vi "track_event.read.vi"(8 "error in":errorcluster, 11 "Track Chunk Core":u8[](array[numeric])) -> (0 "error out":errorcluster, 2 "file events":refnum<class "midi-file-event.lvclass">[](array[class]), 3 "Track Chunk Core Out":u8[](array[numeric]))   [LabVIEW 2020, in "midi-file.lvclass"]
uses:
  midi-file.lvclass
  midi-file-event/midi-file-event.lvclass
  MIDI Meta Events.ctl
  midi-file-event.meta/midi-file-event.meta.lvclass
  C:/code/LabVIEW-MIDI/lv-src/midi-file-event/midi-file-event.lvclass
  midi-file-event.meta/midi-file-event.meta.lvclass/midi-file-event.meta.ctl
  MIDI Messages.ctl
  midi-file-event.midi/midi-file-event.midi.lvclass
  midi-file-event.midi/midi-file-event.midi.lvclass/midi-file-event.midi.ctl
  midi-file-event/midi-file-event.lvclass/midi-file-event.ctl
  midi-file-event.meta/status.set.vi
  midi-file-event.meta/numeric_data.set.vi
  midi-file-event.meta/string_data.set.vi
  midi-file-event.midi/MIDI Messages.set.vi
  midi-file-event.midi/Data1.set.vi
  midi-file-event.midi/Data2.set.vi
  midi-file-event/Delta Tiime.set.vi
  midi-file-event/uid.set.vi
  midi-file.lvclass/midi-file.ctl
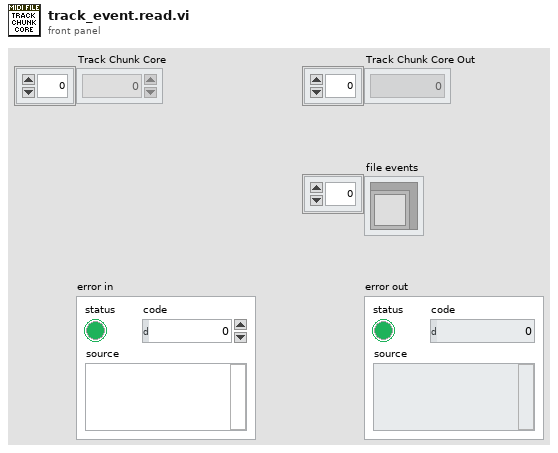
[diagram p1: front panel]
types:
  T1 = typedef "midi-file.lvclass/MIDI Meta Events.ctl" = enum8{"0(0x00)_SequenceNumber", "1(0x01)_TextEvent", "2(0x02)_CopyrightNotice", "3(0x03)_TrackOrSequenceName", "4(0x04)_InstrumentName", "5(0x05)_LyricText", "6(0x06)_MarkerText", "7(0x07)_CuePoint", "8(0x08)_UnassignedMetaEvent", "9(0x09)_UnassignedMetaEvent", "10(0x0A)_UnassignedMetaEvent", "11(0x0B)_UnassignedMetaEvent", "12(0x0C)_UnassignedMetaEvent", "13(0x0D)_UnassignedMetaEvent", "14(0x0E)_UnassignedMetaEvent", "15(0x0F)_UnassignedMetaEvent", "16(0x10)_UnassignedMetaEvent", "17(0x11)_UnassignedMetaEvent", "18(0x12)_UnassignedMetaEvent", "19(0x13)_UnassignedMetaEvent", "20(0x14)_UnassignedMetaEvent", "21(0x15)_UnassignedMetaEvent", "22(0x16)_UnassignedMetaEvent", "23(0x17)_UnassignedMetaEvent", "24(0x18)_UnassignedMetaEvent", "25(0x19)_UnassignedMetaEvent", "26(0x1A)_UnassignedMetaEvent", "27(0x1B)_UnassignedMetaEvent", "28(0x1C)_UnassignedMetaEvent", "29(0x1D)_UnassignedMetaEvent", "30(0x1E)_UnassignedMetaEvent", "31(0x1F)_UnassignedMetaEvent", "32(0x20)_MidiChannelPrefix", "33(0x21)_UnassignedMetaEvent", "34(0x22)_UnassignedMetaEvent", "35(0x23)_UnassignedMetaEvent", "36(0x24)_UnassignedMetaEvent", "37(0x25)_UnassignedMetaEvent", "38(0x26)_UnassignedMetaEvent", "39(0x27)_UnassignedMetaEvent", "40(0x28)_UnassignedMetaEvent", "41(0x29)_UnassignedMetaEvent", "42(0x2A)_UnassignedMetaEvent", "43(0x2B)_UnassignedMetaEvent", "44(0x2C)_UnassignedMetaEvent", "45(0x2D)_UnassignedMetaEvent", "46(0x2E)_UnassignedMetaEvent", "47(0x2F)_EndOfTrack", "48(0x30)_UnassignedMetaEvent", "49(0x31)_UnassignedMetaEvent", "50(0x32)_UnassignedMetaEvent", "51(0x33)_UnassignedMetaEvent", "52(0x34)_UnassignedMetaEvent", "53(0x35)_UnassignedMetaEvent", "54(0x36)_UnassignedMetaEvent", "55(0x37)_UnassignedMetaEvent", "56(0x38)_UnassignedMetaEvent", "57(0x39)_UnassignedMetaEvent", "58(0x3A)_UnassignedMetaEvent", "59(0x3B)_UnassignedMetaEvent", "60(0x3C)_UnassignedMetaEvent", "61(0x3D)_UnassignedMetaEvent", "62(0x3E)_UnassignedMetaEvent", "63(0x3F)_UnassignedMetaEvent", "64(0x40)_UnassignedMetaEvent", "65(0x41)_UnassignedMetaEvent", "66(0x42)_UnassignedMetaEvent", "67(0x43)_UnassignedMetaEvent", "68(0x44)_UnassignedMetaEvent", "69(0x45)_UnassignedMetaEvent", "70(0x46)_UnassignedMetaEvent", "71(0x47)_UnassignedMetaEvent", "72(0x48)_UnassignedMetaEvent", "73(0x49)_UnassignedMetaEvent", "74(0x4A)_UnassignedMetaEvent", "75(0x4B)_UnassignedMetaEvent", "76(0x4C)_UnassignedMetaEvent", "77(0x4D)_UnassignedMetaEvent", "78(0x4E)_UnassignedMetaEvent", "79(0x4F)_UnassignedMetaEvent", "80(0x50)_UnassignedMetaEvent", "81(0x51)_TempoSetting", "82(0x52)_UnassignedMetaEvent", "83(0x53)_UnassignedMetaEvent", "84(0x54)_SMPTEOffset", "85(0x55)_UnassignedMetaEvent", "86(0x56)_UnassignedMetaEvent", "87(0x57)_UnassignedMetaEvent", "88(0x58)_TimeSignature", "89(0x59)_KeySignature", "90(0x5A)_UnassignedMetaEvent", "91(0x5B)_UnassignedMetaEvent", "92(0x5C)_UnassignedMetaEvent", "93(0x5D)_UnassignedMetaEvent", "94(0x5E)_UnassignedMetaEvent", "95(0x5F)_UnassignedMetaEvent", "96(0x60)_UnassignedMetaEvent", "97(0x61)_UnassignedMetaEvent", "98(0x62)_UnassignedMetaEvent", "99(0x63)_UnassignedMetaEvent", "100(0x64)_UnassignedMetaEvent", "101(0x65)_UnassignedMetaEvent", "102(0x66)_UnassignedMetaEvent", "103(0x67)_UnassignedMetaEvent", "104(0x68)_UnassignedMetaEvent", "105(0x69)_UnassignedMetaEvent", "106(0x6A)_UnassignedMetaEvent", "107(0x6B)_UnassignedMetaEvent", "108(0x6C)_UnassignedMetaEvent", "109(0x6D)_UnassignedMetaEvent", "110(0x6E)_UnassignedMetaEvent", "111(0x6F)_UnassignedMetaEvent", "112(0x70)_UnassignedMetaEvent", "113(0x71)_UnassignedMetaEvent", "114(0x72)_UnassignedMetaEvent", "115(0x73)_UnassignedMetaEvent", "116(0x74)_UnassignedMetaEvent", "117(0x75)_UnassignedMetaEvent", "118(0x76)_UnassignedMetaEvent", "119(0x77)_UnassignedMetaEvent", "120(0x78)_UnassignedMetaEvent", "121(0x79)_UnassignedMetaEvent", "122(0x7A)_UnassignedMetaEvent", "123(0x7B)_UnassignedMetaEvent", "124(0x7C)_UnassignedMetaEvent", "125(0x7D)_UnassignedMetaEvent", "126(0x7E)_UnassignedMetaEvent", "127(0x7F)_SequencerSpecificMetaEvent"}
  T2 = typedef "midi-file.lvclass/MIDI Messages.ctl" = enum8{"0(0x00)_UnassignedMidiMessage", "1(0x01)_UnassignedMidiMessage", "2(0x02)_UnassignedMidiMessage", "3(0x03)_UnassignedMidiMessage", "4(0x04)_UnassignedMidiMessage", "5(0x05)_UnassignedMidiMessage", "6(0x06)_UnassignedMidiMessage", "7(0x07)_UnassignedMidiMessage", "8(0x08)_NoteOffEvent", "9(0x09)_NoteOnEvent", "10(0x0A)_PolyphonicKeyPressure", "11(0x0B)_ControlChange", "12(0x0C)_ProgramChange", "13(0x0D)_ChannelPressure", "14(0x0E)_PitchBendChange", "15(0x0F)_SystemExclusive(SysEx)", "16(0x10)_UnassignedMidiMessage", "17(0x11)_UnassignedMidiMessage", "18(0x12)_UnassignedMidiMessage", "19(0x13)_UnassignedMidiMessage", "20(0x14)_UnassignedMidiMessage", "21(0x15)_UnassignedMidiMessage", "22(0x16)_UnassignedMidiMessage", "23(0x17)_UnassignedMidiMessage", "24(0x18)_UnassignedMidiMessage", "25(0x19)_UnassignedMidiMessage", "26(0x1A)_UnassignedMidiMessage", "27(0x1B)_UnassignedMidiMessage", "28(0x1C)_UnassignedMidiMessage", "29(0x1D)_UnassignedMidiMessage", "30(0x1E)_UnassignedMidiMessage", "31(0x1F)_UnassignedMidiMessage", "32(0x20)_UnassignedMidiMessage", "33(0x21)_UnassignedMidiMessage", "34(0x22)_UnassignedMidiMessage", "35(0x23)_UnassignedMidiMessage", "36(0x24)_UnassignedMidiMessage", "37(0x25)_UnassignedMidiMessage", "38(0x26)_UnassignedMidiMessage", "39(0x27)_UnassignedMidiMessage", "40(0x28)_UnassignedMidiMessage", "41(0x29)_UnassignedMidiMessage", "42(0x2A)_UnassignedMidiMessage", "43(0x2B)_UnassignedMidiMessage", "44(0x2C)_UnassignedMidiMessage", "45(0x2D)_UnassignedMidiMessage", "46(0x2E)_UnassignedMidiMessage", "47(0x2F)_UnassignedMidiMessage", "48(0x30)_UnassignedMidiMessage", "49(0x31)_UnassignedMidiMessage", "50(0x32)_UnassignedMidiMessage", "51(0x33)_UnassignedMidiMessage", "52(0x34)_UnassignedMidiMessage", "53(0x35)_UnassignedMidiMessage", "54(0x36)_UnassignedMidiMessage", "55(0x37)_UnassignedMidiMessage", "56(0x38)_UnassignedMidiMessage", "57(0x39)_UnassignedMidiMessage", "58(0x3A)_UnassignedMidiMessage", "59(0x3B)_UnassignedMidiMessage", "60(0x3C)_UnassignedMidiMessage", "61(0x3D)_UnassignedMidiMessage", "62(0x3E)_UnassignedMidiMessage", "63(0x3F)_UnassignedMidiMessage", "64(0x40)_UnassignedMidiMessage", "65(0x41)_UnassignedMidiMessage", "66(0x42)_UnassignedMidiMessage", "67(0x43)_UnassignedMidiMessage", "68(0x44)_UnassignedMidiMessage", "69(0x45)_UnassignedMidiMessage", "70(0x46)_UnassignedMidiMessage", "71(0x47)_UnassignedMidiMessage", "72(0x48)_UnassignedMidiMessage", "73(0x49)_UnassignedMidiMessage", "74(0x4A)_UnassignedMidiMessage", "75(0x4B)_UnassignedMidiMessage", "76(0x4C)_UnassignedMidiMessage", "77(0x4D)_UnassignedMidiMessage", "78(0x4E)_UnassignedMidiMessage", "79(0x4F)_UnassignedMidiMessage", "80(0x50)_UnassignedMidiMessage", "81(0x51)_UnassignedMidiMessage", "82(0x52)_UnassignedMidiMessage", "83(0x53)_UnassignedMidiMessage", "84(0x54)_UnassignedMidiMessage", "85(0x55)_UnassignedMidiMessage", "86(0x56)_UnassignedMidiMessage", "87(0x57)_UnassignedMidiMessage", "88(0x58)_UnassignedMidiMessage", "89(0x59)_UnassignedMidiMessage", "90(0x5A)_UnassignedMidiMessage", "91(0x5B)_UnassignedMidiMessage", "92(0x5C)_UnassignedMidiMessage", "93(0x5D)_UnassignedMidiMessage", "94(0x5E)_UnassignedMidiMessage", "95(0x5F)_UnassignedMidiMessage", "96(0x60)_UnassignedMidiMessage", "97(0x61)_UnassignedMidiMessage", "98(0x62)_UnassignedMidiMessage", "99(0x63)_UnassignedMidiMessage", "100(0x64)_UnassignedMidiMessage", "101(0x65)_UnassignedMidiMessage", "102(0x66)_UnassignedMidiMessage", "103(0x67)_UnassignedMidiMessage", "104(0x68)_UnassignedMidiMessage", "105(0x69)_UnassignedMidiMessage", "106(0x6A)_UnassignedMidiMessage", "107(0x6B)_UnassignedMidiMessage", "108(0x6C)_UnassignedMidiMessage", "109(0x6D)_UnassignedMidiMessage", "110(0x6E)_UnassignedMidiMessage", "111(0x6F)_UnassignedMidiMessage", "112(0x70)_UnassignedMidiMessage", "113(0x71)_UnassignedMidiMessage", "114(0x72)_UnassignedMidiMessage", "115(0x73)_UnassignedMidiMessage", "116(0x74)_UnassignedMidiMessage", "117(0x75)_UnassignedMidiMessage", "118(0x76)_UnassignedMidiMessage", "119(0x77)_UnassignedMidiMessage", "120(0x78)_UnassignedMidiMessage", "121(0x79)_UnassignedMidiMessage", "122(0x7A)_UnassignedMidiMessage", "123(0x7B)_UnassignedMidiMessage", "124(0x7C)_UnassignedMidiMessage", "125(0x7D)_UnassignedMidiMessage", "126(0x7E)_UnassignedMidiMessage", "127(0x7F)_UnassignedMidiMessage"}
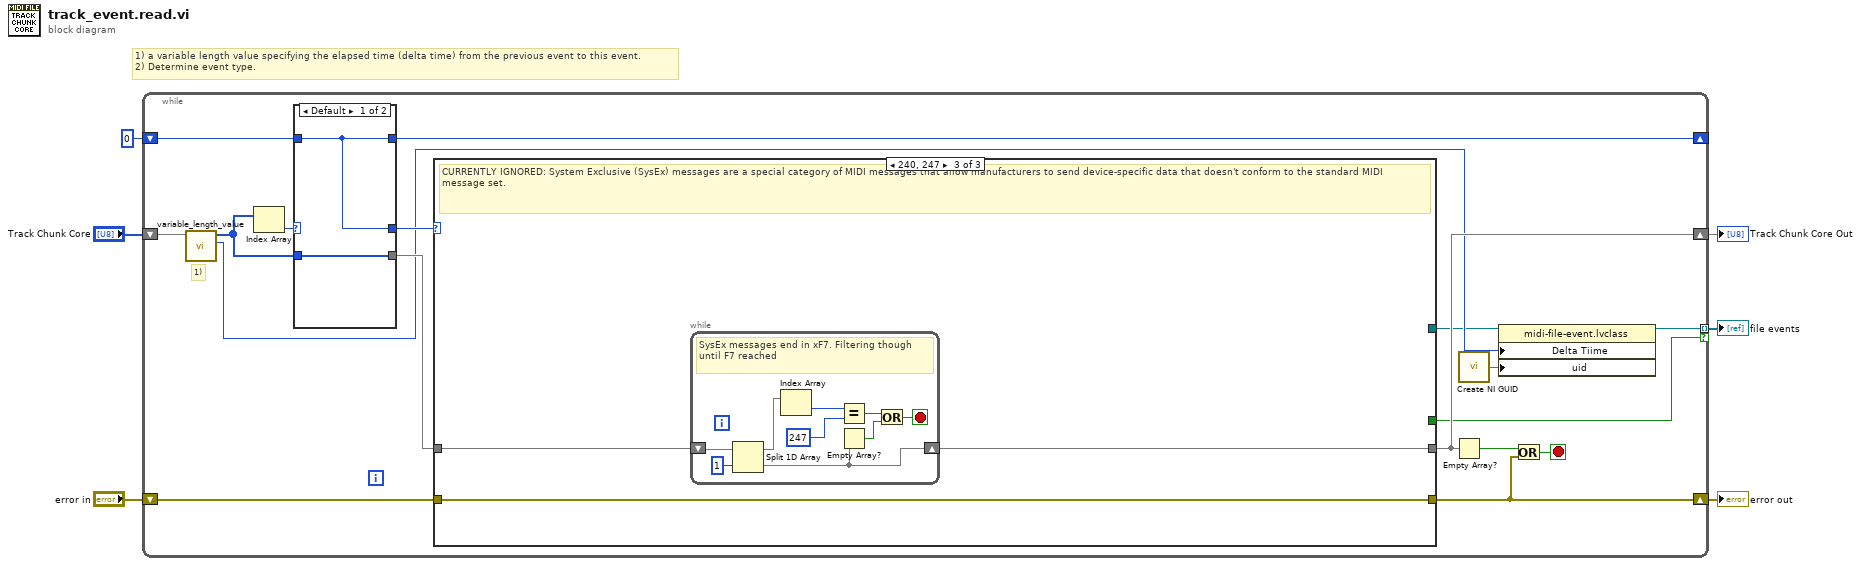
[diagram p0: block diagram]
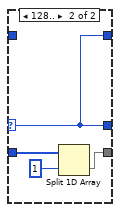
[diagram p2: hidden frame]
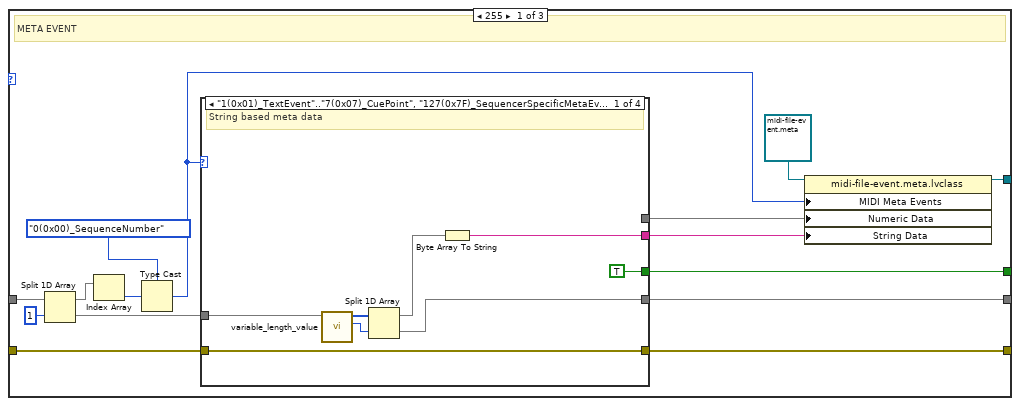
[diagram p3: hidden frame]
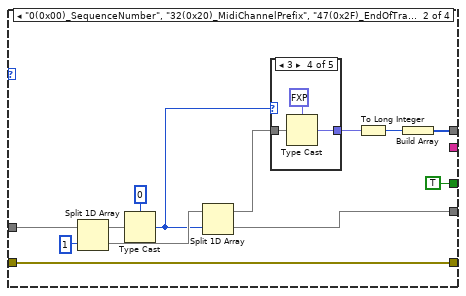
[diagram p4: hidden frame]
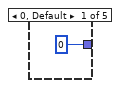
[diagram p5: hidden frame]
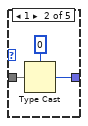
[diagram p6: hidden frame]
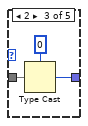
[diagram p7: hidden frame]
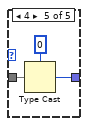
[diagram p8: hidden frame]
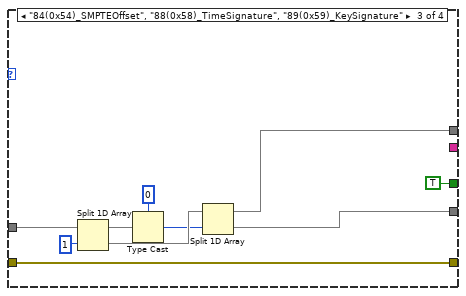
[diagram p9: hidden frame]
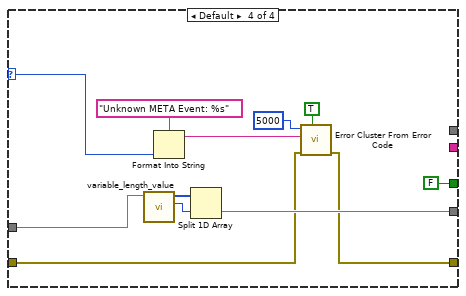
[diagram p10: hidden frame]
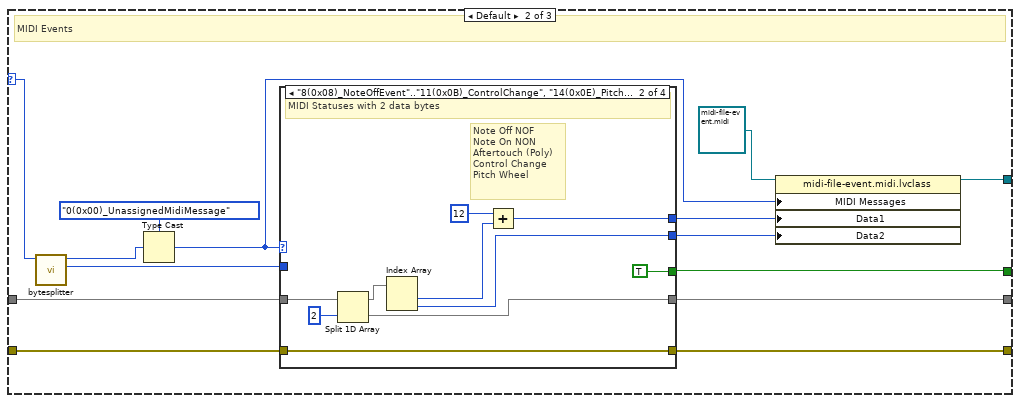
[diagram p11: hidden frame]
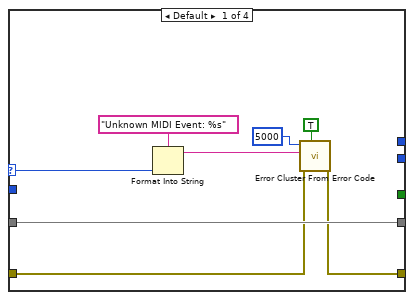
[diagram p12: hidden frame]
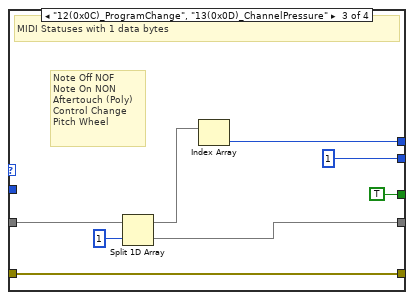
[diagram p13: hidden frame]
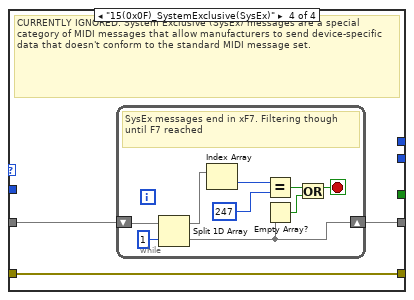
[diagram p14: hidden frame]
diagram:
  # "1) a variable length value specifying the elapsed time (delta time) from the previous event to this event.\n2) Determine event type."
  n1 = while {
    shift-right: [w23] -> w5
    shift-left: "Track Chunk Core" -> [w21]
    tunnel: [w7] -> w1 mode=indexing if=w22
    shift-right: [w18] -> _
    shift-left: u8 0 ("datastream in") -> [w17]
    shift-right: [w13] -> w3
    shift-left: "error in" -> [w14]
    stop <- w11 stop-if-true
    # "1)"
    n2 = call "variable_length_value.vi"("datastream in"=w21) -> ("Variable Length Value"=w10:u32, "datastream out"=w15:u8[])  [unwired: 9 in]
    n3 = Index Array(array=w15) -> (element=w19:u8)  [unwired: 1 in]
    n4 = case shown="Default" w19 {
      selector: w19 -> [_ w29]
      tunnel: [w25 w29] -> w20
      tunnel: [w25 w29] -> w18
      tunnel: w17 -> [w25 _]
      tunnel: [w24 w26] -> w16
      tunnel: w15 -> [w24 w27]
      frame Default {
      }
      frame 128.. {
        n5 = Split 1D Array(array=w27, index=1) -> (second subarray=w26:u8[])  [unwired: 1 out]
      }
    }
    n6 = case shown="240, 247" w20 {
      selector: w20 -> [_ w111 _]
      tunnel: w16 -> [w43 w114 w155]
      tunnel: [w41 w112 w154] -> w23
      tunnel: [w30 w110 _] -> w22
      tunnel: w14 -> [w36 w107 w153]
      tunnel: [w37 w106 w153] -> w13
      tunnel: [w31 w101 _] -> w8
      frame 255 {
        # "META EVENT"
        n7 = Split 1D Array(array=w43, index=1) -> (first subarray=w42:u8[], second subarray=w40:u8[])
        n8 = Index Array(array=w42) -> (element=w39:u8)  [unwired: 1 in]
        n9 = Type Cast(type=MIDI_Meta_Events."0(0x00)_SequenceNumber" ("MIDI Meta Events"), x=w39) -> (*(type *) &x=w34:T1)
        n10 = case shown="\"1(0x01)_TextEvent\"..\"7(0x07)_CuePoint\", \"127(0x7F)_SequencerSpecificMetaEvent\"" w34 {
          selector: w34 -> [_ _ _ w91]
          tunnel: [w50 w60 w82 w97] -> w41
          tunnel: w40 -> [w48 w64 w87 w98]
          tunnel: [w47 _ _ _] -> w33
          tunnel: [_ w57 w81 _] -> w32
          tunnel: [TRUE TRUE TRUE FALSE] -> w30
          tunnel: [w45 w55 w79 w90] -> w37
          tunnel: w36 -> [w45 w55 w79 w89]
          frame "1(0x01)_TextEvent".."7(0x07)_CuePoint", "127(0x7F)_SequencerSpecificMetaEvent" {
            # "String based meta data"
            n11 = call "variable_length_value.vi"("datastream in"=w48) -> ("Variable Length Value"=w52:u32, "datastream out"=w51:u8[])  [unwired: 9 in]
            n12 = Split 1D Array(array=w51, index=w52) -> (first subarray=w49:u8[], second subarray=w50:u8[])
            n13 = Byte Array To String(unsigned byte array=w49) -> (string=w47:string)
          }
          frame "0(0x00)_SequenceNumber", "32(0x20)_MidiChannelPrefix", "47(0x2F)_EndOfTrack", "81(0x51)_TempoSetting" {
            n14 = Split 1D Array(array=w64, index=1) -> (first subarray=w62:u8[], second subarray=w63:u8[])
            n15 = Type Cast(type=u8 0, x=w62) -> (*(type *) &x=w54:u8)
            n16 = Split 1D Array(array=w63, index=w54) -> (first subarray=w59:u8[], second subarray=w60:u8[])
            n17 = case shown="3" w54 {
              tunnel: w59 -> [_ w69 w72 w75 w78]
              tunnel: [0 w68 w71 w74 w77] -> w58
              frame 0, Default {
              }
              frame 1 {
                n18 = Type Cast(type=i8 0, x=w69) -> (*(type *) &x=w68:i8)
              }
              frame 2 {
                n19 = Type Cast(type=i16 0, x=w72) -> (*(type *) &x=w71:i16)
              }
              frame 3 {
                n20 = Type Cast(type=fxp<+/-,24,24> 0.0, x=w75) -> (*(type *) &x=w74:fxp<+/-,24,24>)
              }
              frame 4 {
                n21 = Type Cast(type=i64 0, x=w78) -> (*(type *) &x=w77:i64)
              }
            }
            n22 = To Long Integer(number=w58) -> (32bit integer=w53:i32)
            n23 = Build Array(w53) -> (w57:i32[])
          }
          frame "84(0x54)_SMPTEOffset", "88(0x58)_TimeSignature", "89(0x59)_KeySignature" {
            n24 = Split 1D Array(array=w87, index=1) -> (first subarray=w85:u8[], second subarray=w86:u8[])
            n25 = Type Cast(type=u8 0, x=w85) -> (*(type *) &x=w83:u8)
            n26 = Split 1D Array(array=w86, index=w83) -> (first subarray=w81:u8[], second subarray=w82:u8[])
          }
          frame Default {
            n27 = call "variable_length_value.vi"("datastream in"=w98) -> ("Variable Length Value"=w100:u32, "datastream out"=w99:u8[])  [unwired: 9 in]
            n28 = Format Into String(format string="Unknown META Event: %s", w91) -> (resulting string=w93:string)  [unwired: 2 in, 1 out]
            n29 = Split 1D Array(array=w99, index=w100) -> (second subarray=w97:u8[])  [unwired: 1 out]
            n30 = call <vilib>:"Error Cluster From Error Code.vi"("show call chain? (False)"=TRUE, "error in (no error)"=w89, "error message (\"\")"=w93, "error code (0)"=5000) -> ("error out"=w90:errorcluster)  [unwired: 5 in]
          }
        }
        n31 = property class="midi-file-event.meta.lvclass"(reference=refnum<class "midi-file-event.meta.lvclass"> refnum ("midi-file-event.meta.lvclass"), "MIDI Meta Events"=w34, "Numeric Data"=w32, "String Data"=w33) -> (reference out=w31:refnum<class "midi-file-event.meta.lvclass">)  [unwired: 1 in, 1 out]
      }
      frame Default {
        # "MIDI Events"
        n32 = call "bytesplitter.vi"("Byte"=w111) -> ("Low Nibble"=w113:u8, "High Nibble"=w108:u8)  [unwired: 9 in]
        n33 = Type Cast(type=MIDI_Messages."0(0x00)_UnassignedMidiMessage" ("MIDI Messages"), x=w108) -> (*(type *) &x=w102:T2)
        n34 = case shown="\"8(0x08)_NoteOffEvent\"..\"11(0x0B)_ControlChange\", \"14(0x0E)_PitchBendChange\"" w102 {
          selector: w102 -> [w118 _ _ _]
          tunnel: w114 -> [w122 w131 w139 w143]
          tunnel: w113 -> [_ _ _ _]
          tunnel: [w122 w130 w138 w142] -> w112
          tunnel: [_ TRUE TRUE _] -> w110
          tunnel: w107 -> [w117 w125 w135 w141]
          tunnel: [w116 w125 w135 w141] -> w106
          tunnel: [_ w124 w134 _] -> w104
          tunnel: [_ w123 u8 1 _] -> w103
          frame Default {
            n35 = Format Into String(format string="Unknown MIDI Event: %s", w118) -> (resulting string=w119:string)  [unwired: 2 in, 1 out]
            n36 = call <vilib>:"Error Cluster From Error Code.vi"("show call chain? (False)"=TRUE, "error in (no error)"=w117, "error message (\"\")"=w119, "error code (0)"=5000) -> ("error out"=w116:errorcluster)  [unwired: 5 in]
          }
          frame "8(0x08)_NoteOffEvent".."11(0x0B)_ControlChange", "14(0x0E)_PitchBendChange" {
            # "Note Off NOF\nNote On NON\nAftertouch (Poly)\nControl Change\nPitch Wheel"
            # "MIDI Statuses with 2 data bytes"
            n37 = Split 1D Array(array=w131, index=2) -> (first subarray=w129:u8[], second subarray=w130:u8[])
            n38 = Index Array(array=w129) -> (element #1=w127:u8, element #2=w123:u8)  [unwired: 2 in]
            n39 = Add(x=u8 12 ("y"), y=w127) -> (x+y=w124:u8)
          }
          frame "12(0x0C)_ProgramChange", "13(0x0D)_ChannelPressure" {
            # "Note Off NOF\nNote On NON\nAftertouch (Poly)\nControl Change\nPitch Wheel"
            # "MIDI Statuses with 1 data bytes"
            n40 = Split 1D Array(array=w139, index=1) -> (first subarray=w137:u8[], second subarray=w138:u8[])
            n41 = Index Array(array=w137) -> (element=w134:u8)  [unwired: 1 in]
          }
          frame "15(0x0F)_SystemExclusive(SysEx)" {
            # "CURRENTLY IGNORED: System Exclusive (SysEx) messages are a special category of MIDI messages that allow manufacturers to send device-specific data that doesn't conform to the standard MIDI message set."
            n42 = while {
              shift-right: [w146] -> w142
              shift-left: w143 -> [w152]
              stop <- w144 stop-if-true
              # "SysEx messages end in xF7. Filtering though until F7 reached"
              n43 = Split 1D Array(array=w152, index=1) -> (first subarray=w150:u8[], second subarray=w146:u8[])
              n44 = Index Array(array=w150) -> (element=w149:u8)  [unwired: 1 in]
              n45 = Equal?(x=w149, y=u8 247) -> (x = y?=w147:bool)
              n46 = Empty Array?(array=w146) -> (empty?=w145:bool)
              n47 = Or(x=w147, y=w145) -> (x .or. y?=w144:bool)
            }
          }
        }
        n48 = property class="midi-file-event.midi.lvclass"(reference=refnum<class "midi-file-event.midi.lvclass"> refnum ("midi-file-event.midi.lvclass"), "MIDI Messages"=w102, "Data1"=w104, "Data2"=w103) -> (reference out=w101:refnum<class "midi-file-event.midi.lvclass">)  [unwired: 1 in, 1 out]
      }
      frame 240, 247 {
        # "CURRENTLY IGNORED: System Exclusive (SysEx) messages are a special category of MIDI messages that allow manufacturers to send device-specific data that doesn't conform to the standard MIDI message set."
        n49 = while {
          shift-right: [w158] -> w154
          shift-left: w155 -> [w164]
          stop <- w156 stop-if-true
          # "SysEx messages end in xF7. Filtering though until F7 reached"
          n50 = Split 1D Array(array=w164, index=1) -> (first subarray=w162:u8[], second subarray=w158:u8[])
          n51 = Index Array(array=w162) -> (element=w161:u8)  [unwired: 1 in]
          n52 = Equal?(x=w161, y=u8 247) -> (x = y?=w159:bool)
          n53 = Empty Array?(array=w158) -> (empty?=w157:bool)
          n54 = Or(x=w159, y=w157) -> (x .or. y?=w156:bool)
        }
      }
    }
    n55 = Empty Array?(array=w23) -> (empty?=w12:bool)
    n56 = call <vilib>:"Create NI GUID.vi"() -> ("NI GUID"=w9:string)
    n57 = property class="midi-file-event.lvclass"(reference=w8, "Delta Tiime"=w10, "uid"=w9) -> (reference out=w7:refnum<class "midi-file-event.lvclass">)  [unwired: 1 in, 1 out]
    n58 = Or(x=w12, y=w13) -> (x .or. y?=w11:bool)
  }
  "Track Chunk Core Out" <- w5
  "error out" <- w3
  "file events" <- w1
